vi "Get_SoundFile_Binary.vi"(8 "error in (no error)":errorcluster, 10 "Sound File Name":string, 11 "Session In":T1) -> (0 "error out":errorcluster, 2 "Binary String":string, 3 "Session Out":T1)   [LabVIEW 2018, in "MerriamWebsterJSON.lvlib"]
uses:
  MerriamWebsterJSON.lvlib
  <vilib>/httpClient/ClientHandle.ctl
  <vilib>/httpClient/LabVIEWHTTPClient.lvlib
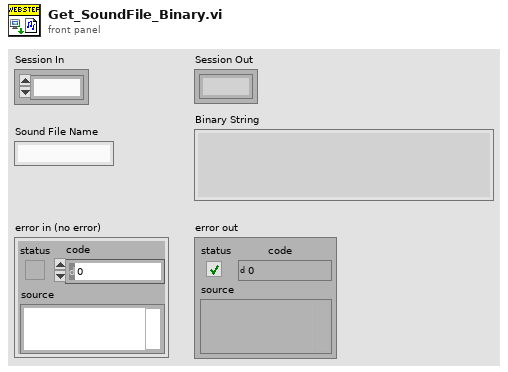
[diagram p1: front panel]
types:
  T1 = typedef "LabVIEWHTTPClient.lvlib/ClientHandle.ctl" = refnum<k1>
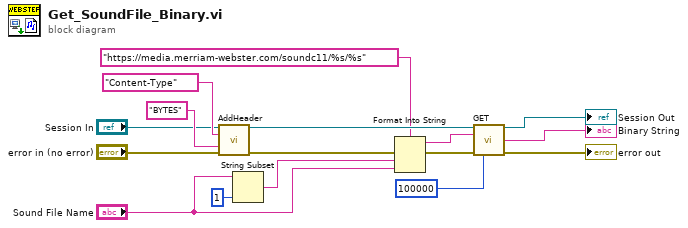
[diagram p0: block diagram]
diagram:
  n1 = call <vilib>:"AddHeader.vi"("client handle"="Session In", "header"="Content-Type", "value"="BYTES", "error in (no error)"="error in (no error)") -> ("client handle out"=w13:T1, "error out"=w8:errorcluster)  [unwired: 10 in]
  n2 = String Subset(string="Sound File Name", length (rest)=1 ("length (rest)")) -> (substring=w9:string)  [unwired: 1 in]
  n3 = Format Into String(format string="https://media.merriam-webster.com/soundc11/%s/%s", error in=w8, w9, "Sound File Name") -> (resulting string=w5:string, error out=w7:errorcluster)  [unwired: 1 in]
  n4 = call <vilib>:"GET.vi"("client handle"=w13, "url"=w5, "error in (no error)"=w7, "timeout (10000)"=100000) -> ("client handle out"=→"Session Out":T1, "body"=→"Binary String":string, "error out"=→"error out":errorcluster)  [unwired: 8 in, 1 out]
